vi "Manual.vi"(8 "error in (no error)":errorcluster, 10 "event source":refnum<user-event>, 11 "String":string) -> (0 "error out":errorcluster)   [LabVIEW 2026]
uses:
  <vilib>/Handler Framework/Handler Framework.lvlib
  <vilib>/Handler Framework/CmdQueue/Enqueue Single.vi
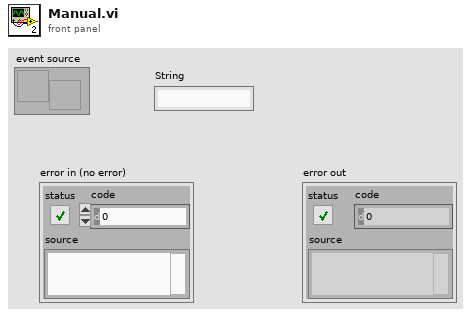
[diagram p1: front panel]
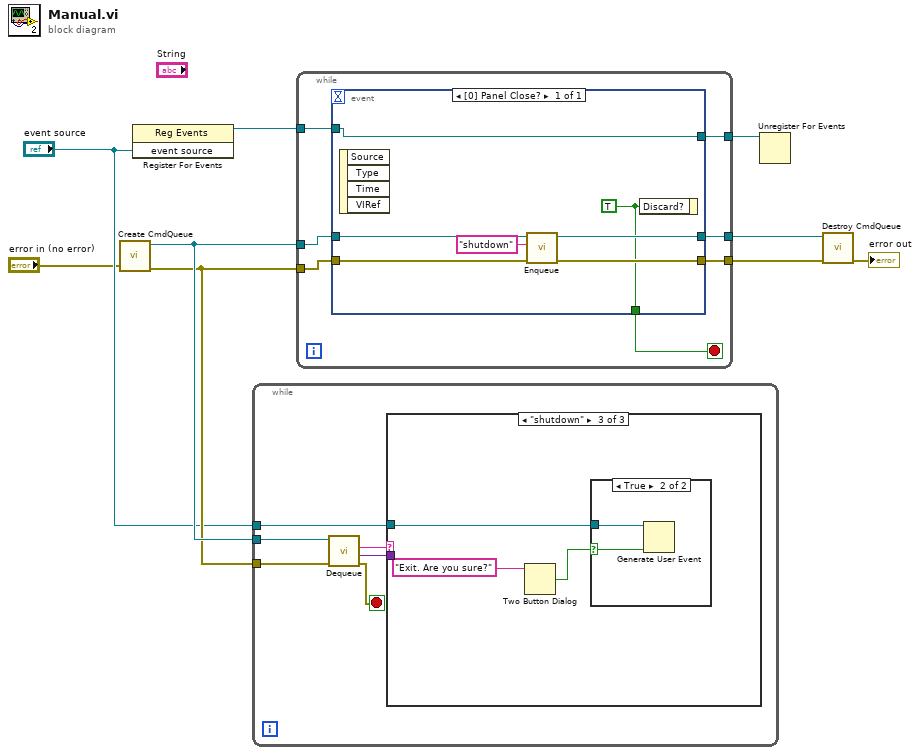
[diagram p0: block diagram]
diagram:
  n1 = call <vilib>:"Create CmdQueue.vi"("error in (no error)"="error in (no error)") -> ("error out"=w6:errorcluster, "CmdQueue out"=w7:refnum<queue>)  [unwired: 9 in]
  n2 = register-events("event source") -> (reference out=w5:refnum<event-registration>)  [unwired: 2 in, 1 out]
  n3 = while {
    tunnel: w7 -> [w15]
    tunnel: w6 -> [w11]
    tunnel: "event source" -> [w10]
    stop <- w12 stop-if-true
    n4 = call <vilib>:"Dequeue.vi"("error in (no error)"=w11, "CmdQueue in"=w15) -> ("error out"=w12:errorcluster, "value"=w13:variant, "cmd"=w14:string)  [unwired: 5 in, 2 out]
    n5 = case shown="\"shutdown\"" w14 {
      tunnel: w13 -> [_ _ _]
      tunnel: w10 -> [_ _ w16]
      frame "False", Default {
      }
      frame "init" {
      }
      frame "shutdown" {
        n6 = Two Button Dialog(message="Exit. Are you sure?") -> (T button?=w17:bool)  [unwired: 2 in]
        n7 = case shown="True" w17 {
          selector: w17 -> [_ w19]
          tunnel: w16 -> [_ w20]
          frame False {
          }
          frame True {
            n8 = Generate User Event(user event=w20, event data cluster=w19) -> ()  [unwired: 2 in, 2 out]
          }
        }
      }
    }
  }
  n9 = while {
    tunnel: w7 -> [w27]
    tunnel: [w26] -> w9
    tunnel: w6 -> [w25]
    tunnel: [w24] -> w8
    tunnel: w5 -> [w22]
    tunnel: [w21] -> w4
    stop <- w23 stop-if-true
    n10 = event shown="[0] Panel Close?" {
      selector: _ -> [_]
      dyn-events: _ -> [_]
      timeout: _ -> [_]
      tunnel: w27 -> [w34]
      tunnel: [w33] -> w26
      tunnel: w25 -> [w32]
      tunnel: [w31] -> w24
      tunnel: [w29] -> w23
      tunnel: w22 -> [w28]
      tunnel: [w28] -> w21
      event Panel Close? {
        w29 = TRUE ("Discard?")
        n11 = event-data() -> ()  [unwired: 1 in, 4 out]
        n12 = call-poly <vilib>:"Enqueue.vi"("error in (no error)"=w32, "Command"="shutdown", "CmdQueue in"=w34) -> ("error out"=w31:errorcluster, "CmdQueue out"=w33:refnum<queue>)  [unwired: 7 in]
        n13 = event-data("Discard?"=w29) -> ()  [unwired: 1 in, 1 out]
      }
    }
  }
  n14 = Unregister For Events(event registration refnum=w4) -> ()  [unwired: 1 in, 1 out]
  n15 = call <vilib>:"Destroy CmdQueue.vi"("error in (no error)"=w8, "CmdQueue in"=w9) -> ("error out"=→"error out":errorcluster)  [unwired: 9 in]
